vi "SetActiveMarker.vi"(8 "error in (no error)":errorcluster, 11 "Keysight44xx in":refnum<class "Keysight44xx.lvclass">) -> (0 "error out":errorcluster, 3 "Keysight44xx out":refnum<class "Keysight44xx.lvclass">)   [LabVIEW 2018, in "SpecAnPlugins.lvlib" / "Keysight44xx.lvclass"]
doc: "This VI selects one of the available markers, and makes it the active marker. The active marker must be enabled using Configure Marker Enabled VI/method before it can be used for most marker operations. The Active Marker can be set between 1 and Number Of Markers."
uses:
  Keysight44xx.lvclass
  C:/Users/ico/Documents/Projects/NistPluggableModules/SpecAn/SpecAnPlugins/SpecAnBaseClass/SpecAnBase.lvclass
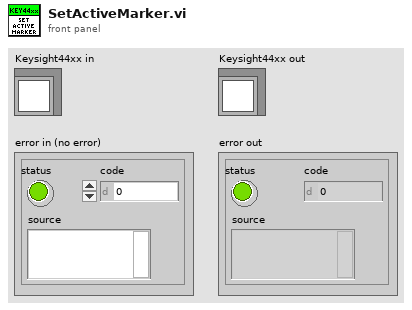
[diagram p1: front panel]
types:
  T1 = typedef "SpecAnPlugins.lvlib/SpecAnBase.lvclass/Acquisition.ctl" = cluster{"Handle":string, "Connected":bool, "Enabled":bool, "SweepModeContinuous":bool, "NumberOfSweeps":i32, "DetectorTypeAuto":bool, "DetectorType":i32, "VerticalScale":i32, "MaximumTime(seconds)":dbl}
  T2 = typedef "SpecAnPlugins.lvlib/SpecAnBase.lvclass/Markers.ctl" = cluster{"MarkerEnabled":bool, "MarkerThreshold":dbl, "PeakExcursion":dbl, "SignalTrackEnabled":bool, "MarkerPosition":dbl, "Instrument Setting (Frequency Center)":i32, "Marker search (Minimum)":i32, "ActiveMarker":string, "MarkerFrequencyCounter":bool, "FrequencyCounterResolution":dbl}
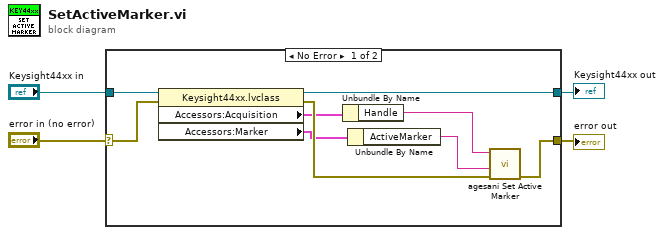
[diagram p0: block diagram]
diagram:
  n1 = case shown="No Error" "error in (no error)" {
    selector: "error in (no error)" -> [w12 w15]
    tunnel: "Keysight44xx in" -> [w13 w14]
    tunnel: [w6 w15] -> w2
    tunnel: [w11 w14] -> w1
    frame No Error {
      n2 = property class="Keysight44xx.lvclass"(reference=w13, error in=w12) -> (reference out=w11:refnum<class "Keysight44xx.lvclass">, error out=w10:errorcluster, "Accessors:Acquisition"=w9:T1, "Accessors:Marker"=w8:T2)
      n3 = Unbundle By Name(w9) -> ("Handle"=w7:string)
      n4 = Unbundle By Name(w8) -> ("ActiveMarker"=w5:string)
      n5 = call <instrlib>:"agesani Set Active Marker.vi"("error in (no error)"=w10, "active marker (\"MARKER1\")"=w5, "instrument handle"=w7) -> ("error out"=w6:errorcluster)  [unwired: 7 in, 1 out]
    }
    frame Error {
    }
  }
  "error out" <- w2
  "Keysight44xx out" <- w1
